vi "Start Logger.vi"(8 "error in (no error)":errorcluster, 11 "Measure Controller in":refnum<class "Measure Controller.lvclass">) -> (0 "error out":errorcluster, 2 "File Path":path, 3 "Measure Controller out":refnum<class "Measure Controller.lvclass">)   [LabVIEW 2015, in "Measure Controller.lvclass"]
uses:
  Measure Controller.lvclass
  Measure Controller.lvclass/Measure Controller.ctl
  Results/Acquired Result/Acquired Result.lvclass
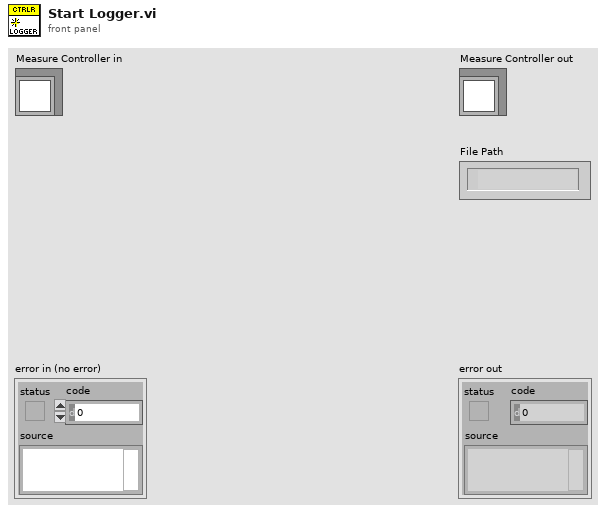
[diagram p1: front panel]
types:
  T1 = enum16{"open", "open or create", "create or replace", "create", "open (read-only)"}
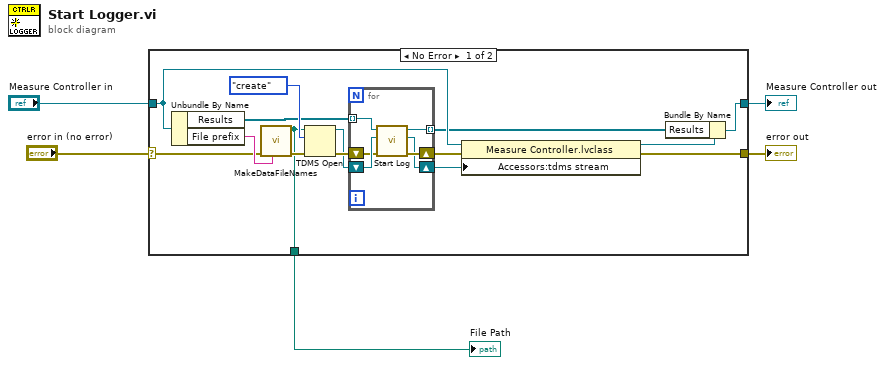
[diagram p0: block diagram]
diagram:
  n1 = case shown="No Error" "error in (no error)" {
    selector: "error in (no error)" -> [w15 w28]
    tunnel: [w14 w28] -> w4
    tunnel: [w12 w27] -> w2
    tunnel: "Measure Controller in" -> [w17 w27]
    tunnel: [w6 _] -> w1
    frame No Error {
      n2 = Unbundle By Name(w17) -> ("Results"=w8:refnum<class "Acquired Result.lvclass">[], "File prefix"=w16:string)
      n3 = call "MakeDataFileNames.vi"("File Prefix"=w16, "Error In"=w15) -> ("Error Out"=w20:errorcluster, "Data File  Path"=w6:path)  [unwired: 6 in, 2 out]
      n4 = TDMS Open(8:w20, 10:T1."create" ("operation (0:open)"), 11:w6) -> (0:w13:errorcluster, 3:w7:refnum<k34>)  [unwired: 4 in]
      n5 = for {
        tunnel: w8 -> [w26] mode=indexing
        shift-right: [w23] -> w10
        shift-left: w13 -> [w24]
        shift-right: [w22] -> w9
        shift-left: w7 -> [w25]
        tunnel: [w21] -> w11 mode=indexing
        n6 = call-dynamic "Start Log.vi"("error in (no error)"=w24, "tdms file"=w25, "Acquired Result in"=w26) -> ("error out"=w23:errorcluster, "tdms file out"=w22:refnum<k34>, "Acquired Result out"=w21:refnum<class "Acquired Result.lvclass">)  [unwired: 6 in]
      }
      n7 = property class="Measure Controller.lvclass"(reference=w17, error in=w10, "Accessors:tdms stream"=w9) -> (reference out=w18:refnum<class "Measure Controller.lvclass">, error out=w14:errorcluster)
      n8 = Bundle By Name(cluster=w18, "Results"=w11) -> (w12:refnum<class "Measure Controller.lvclass">)
    }
    frame Error {
    }
  }
  "error out" <- w4
  "Measure Controller out" <- w2
  "File Path" <- w1
